vi "诊断标定3 - 副本.vi"(8 "CAN端口":u16(ring), 9 "设备索引号":u16(ring), 10 "CAN卡类型":u32(ring)=21) -> ()   [LabVIEW 2013] (continued)
            tunnel: w99 -> [_ w107]
            frame #0 {
              n49 = case shown="假" w102 {
                tunnel: w101 -> [w104 _]
                frame False {
                  n50 = Build Array("文件格式错误") -> (w105:string[])
                  n51 = call "表格编辑.vi"("新元素/子数组"=w105, "活动单元格:单元格背景色"=u32 16711680, "MCListbox引用句柄"=w104) -> ()  [unwired: 9 out]
                }
                frame True {
                }
              }
            }
            frame #1 {
              n52 = case shown="假" w107 {
                tunnel: w108 -> [w110 _]
                frame False {
                  n53 = Build Array("文件MD5码验证错误") -> (w111:string[])
                  n54 = call "表格编辑.vi"("新元素/子数组"=w111, "活动单元格:单元格背景色"=u32 16711680, "MCListbox引用句柄"=w110) -> ()  [unwired: 9 out]
                }
                frame True {
                }
              }
            }
          }
          n55 = call <vilib>:"Unset Busy.vi"() -> ()  [unwired: 11 in, 1 out]
        }
        frame True {
          n56 = stacked-sequence {
            seq-local: [w119 _ _ _] -> [_ w347 w441 _]
            seq-local: [w117 _ _ _] -> [_ w325 _ _]
            tunnel: w114 -> [w115 _ _ _]
            tunnel: w113 -> [w132 _ _ w468]
            frame #0 {
              w116 = string[][] []
              w129 = "总信息" ("section")
              n57 = local write "路径"(w115) -> ()
              n58 = call <vilib>:"Open Config Data.vi"("create file if necessary (T)"=FALSE, "configuration file path"=w115) -> ("error out"=w120:errorcluster, "refnum"=w119:T19)  [unwired: 7 in, 1 out]
              n59 = call <vilib>:"Get Key Names.vi"("section"=w129, "error in (no error)"=w120, "refnum"=w119) -> ("key names"=w128:string[], "refnum out"=w130:T19)  [unwired: 5 in, 2 out]
              n60 = for {
                tunnel: w130 -> [w136]
                tunnel: w129 -> [w135]
                tunnel: w128 -> [w134] mode=indexing
                tunnel: [w133] -> w125 mode=indexing
                n61 = call-poly <vilib>:"Read Key.vi"("section"=w135, "key"=w134, "refnum"=w136) -> ("value"=w133:string)  [unwired: 5 in, 3 out]
              }
              n62 = Index Array(array=w125) -> (element #1=w118:string, element #2=w123:string)  [unwired: 2 in]
              n63 = Decimal String To Number(string=w118) -> (number=w117:i32)  [unwired: 2 in, 1 out]
              n64 = Concatenate Strings("正在读取" ("字符串"), w123, "的配置文件" ("字符串")) -> (w121:string)
              n65 = Build Array(w121) -> (w126:string[])
              n66 = call "表格编辑.vi"("新元素/子数组"=w126, "活动单元格:单元格背景色"=u32 6618880, "MCListbox引用句柄"=w132) -> ()  [unwired: 9 out]
              n67 = local write "项目信息"(w116) -> ()
              n68 = local write "项目信息 2"(w116) -> ()
            }
            frame #1 {
              w307 = 20 ("长度")
              w348 = "主板" ("section")
              n69 = call <vilib>:"Get Key Names.vi"("section"=w348, "refnum"=w347) -> ("key names"=w149:string[], "refnum out"=w349:T19)  [unwired: 6 in, 2 out]
              n70 = for {
                tunnel: w349 -> [w361]
                tunnel: w348 -> [w360]
                tunnel: w149 -> [w359] mode=indexing
                tunnel: [w358] -> w148 mode=indexing
                n71 = call-poly <vilib>:"Read Key.vi"("section"=w360, "key"=w359, "refnum"=w361) -> ("value"=w358:string)  [unwired: 5 in, 3 out]
              }
              n72 = Search 1D Array(1D array=w149, element="总电压过高一级" ("元素"), start index (0)=0 ("开始索引(0)")) -> (index of element=w229:i32)
              n73 = Search 1D Array(1D array=w149, element="风机开启温度" ("元素"), start index (0)=w229) -> (index of element=w220:i32)
              n74 = Search 1D Array(1D array=w149, element="电池串联" ("元素"), start index (0)=w220) -> (index of element=w218:i32)
              n75 = Decrement(x=w229) -> (x-1=w346:i32)
              n76 = Array Subset(array=w149, index=1 ("索引"), length=w346) -> (w194:string[])
              n77 = Array Subset(array=w148, index=1 ("索引"), length=w346) -> (w191:string[])
              n78 = Delete From Array(array=w191, length=7 ("长度"), index=0 ("索引")) -> (deleted portion=w188:string[], array with subset deleted=w138:string[])
              n79 = Delete From Array(array=w194, length=7 ("长度"), index=0 ("索引")) -> (array with subset deleted=w147:string[])  [unwired: 1 out]
              n80 = Search 1D Array(1D array=w149, element="分流器型号" ("元素")) -> (index of element=w152:i32)  [unwired: 1 in]
              n81 = Index Array(array=w148, index=0 ("索引")) -> (element=w322:string)
              n82 = Decimal String To Number(string=w322) -> (number=w139:i32)  [unwired: 2 in, 1 out]
              n83 = Search 1D Array(1D array=w147, element="主板电池节数" ("元素")) -> (index of element=w313:i32)  [unwired: 1 in]
              n84 = Search 1D Array(1D array=w147, element="主板温度起始值" ("元素")) -> (index of element=w310:i32)  [unwired: 1 in]
              n85 = Search 1D Array(1D array=w147, element="第一个保险通道" ("元素")) -> (index of element=w309:i32)  [unwired: 1 in]
              n86 = Search 1D Array(1D array=w147, element="主板温度个数" ("元素")) -> (index of element=w311:i32)  [unwired: 1 in]
              n87 = Search 1D Array(1D array=w147, element="主板电压起始值" ("元素")) -> (index of element=w312:i32)  [unwired: 1 in]
              n88 = Search 1D Array(1D array=w147, element="第1通道电压个数" ("元素")) -> (index of element=w308:i32)  [unwired: 1 in]
              n89 = Index Array(array=w148, index=w152) -> (element=w151:string)
              n90 = for {
                N: 4 -> [_]
                tunnel: w188 -> [w357] mode=indexing
                tunnel: [w356] -> w337 mode=indexing
                n91 = Fract/Exp String To Number(string=w357) -> (number=w356:dbl)  [unwired: 3 in, 1 out]
              }
              n92 = Increment(x=w139) -> (x+1=w321:i32)
              n93 = Increment(x=w139) -> (x+1=w306:i32)
              n94 = Increment(x=w139) -> (x+1=w319:i32)
              n95 = Increment(x=w139) -> (x+1=w320:i32)
              n96 = global write "读配置文件全局.vi" "从板个数"(w139) -> ()
              n97 = local write "从板个数"(w139) -> ()
              n98 = Decimal String To Number(string=w151) -> (number=w150:i32)  [unwired: 2 in, 1 out]
              n99 = Index Array(array=w188, index #1=4 ("索引"), index #2=5 ("索引"), index #3=6 ("索引")) -> (element #1=w328:string, element #2=w327:string, element #3=w326:string)
              n100 = Index Array(array=w337) -> (element #1=w335:dbl, element #2=w334:dbl, element #3=w333:dbl, element #4=w332:dbl)  [unwired: 4 in]
              n101 = global write "EV05全局变量1.vi" "分流器型号"(w150) -> ()
              n102 = Array Subset(array=w138, index=w313, length=w321) -> (w305:string[])
              n103 = Array Subset(array=w138, index=w312, length=w320) -> (w303:string[])
              n104 = Array Subset(array=w138, index=w311, length=w319) -> (w302:string[])
              n105 = Array Subset(array=w138, index=w310, length=w306) -> (w301:string[])
              n106 = Array Subset(array=w138, index=w309, length=20 ("长度")) -> (w300:string[])
              n107 = Array Subset(array=w138, index=w308, length=w307) -> (w304:string[])
              n108 = Multiply(x=w139, y=2) -> (x*y=w140:i32)
              n109 = control-ref of="项目信息2"() -> (w340:refnum<vi>)
              n110 = Array Subset(array=w138, index=0 ("索引"), length=w140) -> (w137:string[])
              n111 = Insert Into Array(array=w305, new element #1=w304, new element #2=w303, new element #3=w302, new element #4=w301, new element #5=w300) -> ()  [unwired: 1 in, 1 out]
              n112 = property class="Clust (严格)"(reference=w340) -> (reference out=w338:refnum<vi>, "Value"=w339:T9)  [unwired: 1 in, 1 out]
              n113 = Multiply(x=w139, y=2) -> (x*y=w144:i32)
              n114 = Array Subset(array=w147, index=w313, length=w306) -> (w178:string[])
              n115 = Array Subset(array=w147, index=w312, length=w306) -> (w176:string[])
              n116 = Array Subset(array=w147, index=w311, length=w306) -> (w175:string[])
              n117 = Array Subset(array=w147, index=w310) -> (w174:string[])  [unwired: 1 in]
              n118 = Array Subset(array=w147, index=w309, length=w307) -> (w173:string[])
              n119 = Array Subset(array=w147, index=w308, length=w307) -> (w177:string[])
              n120 = Array Subset(array=w147, index=0 ("索引"), length=w144) -> (w143:string[])
              n121 = global write "读配置文件全局.vi" "表格输入"(w137) -> ()
              n122 = Build Array(w143, w137) -> (w299:string[][])
              n123 = Bundle(cluster=w339, "电池额定容量(A)"=w335, "使用者"=w325, "电池实际容量(A)"=w334, "车架(牌)号"=w327, "配置文件版本"=w326, "SOH(%)"=w332, "SOC(%)"=w333, "产品编号"=w328) -> (w165:T9)  [unwired: 1 in]
              n124 = Transpose 2D Array(2D array=w299) -> (transposed array=w166:string[][])
              n125 = Multiply(x=w139, y=4) -> (x*y=w170:i32)
              n126 = Insert Into Array(array=w178, new element #1=w177, new element #2=w176, new element #3=w175, new element #4=w174, new element #5=w173) -> (w172:string[])  [unwired: 1 in]
              n127 = Add(x=w170, y=44) -> (x+y=w168:i32)
              n128 = local write "项目信息"(w166) -> ()
              n129 = property class="Clust (严格)"(reference=w338, "Value"=w165) -> ()  [unwired: 1 in, 2 out]
              n130 = global write "读配置文件全局.vi" "项目信息"(w165) -> ()
              n131 = Array Subset(array=w148, index=w218, length=15 ("长度")) -> (w156:string[])
              n132 = Array Subset(array=w172, index=0 ("索引"), length=w168) -> ()  [unwired: 1 out]
              n133 = Array Subset(array=w148, index=w220, length=15 ("长度")) -> (w225:string[])
              n134 = Delete From Array(array=w156, length=4 ("长度"), index=6 ("索引")) -> (deleted portion=w212:string[], array with subset deleted=w211:string[])
              n135 = for {
                tunnel: w225 -> [w353] mode=indexing
                tunnel: [w352] -> w224 mode=indexing
                n136 = Fract/Exp String To Number(string=w353) -> (number=w352:dbl)  [unwired: 3 in, 1 out]
              }
              n137 = for {
                tunnel: w211 -> [w351] mode=indexing
                tunnel: [w350] -> w210 mode=indexing
                n138 = Fract/Exp String To Number(string=w351) -> (number=w350:dbl)  [unwired: 3 in, 1 out]
              }
              n139 = Array Subset(array=w148, index=w229, length=51 ("长度")) -> (w298:string[])
              n140 = for {
                tunnel: w298 -> [w355] mode=indexing
                tunnel: [w354] -> w297 mode=indexing
                n141 = Fract/Exp String To Number(string=w355) -> (number=w354:dbl)  [unwired: 3 in, 1 out]
              }
              n142 = Index Array(array=w210) -> (element #1=w205:dbl, element #2=w204:dbl, element #3=w203:dbl, element #4=w202:dbl, element #5=w201:dbl, element #6=w200:dbl, element #7=w199:dbl, element #8=w198:dbl, element #9=w197:dbl, element #10=w196:dbl, element #11=w195:dbl)  [unwired: 11 in]
              n143 = Delete From Array(array=w224, length=7 ("长度"), index=0 ("索引")) -> (deleted portion=w161:dbl[], array with subset deleted=w222:dbl[])
              n144 = Delete From Array(array=w297, length=17 ("长度"), index=0 ("索引")) -> (deleted portion=w158:dbl[], array with subset deleted=w294:dbl[])
              n145 = Array To Cluster(array=w161) -> (cluster=w223:T20)
              n146 = global write "读配置文件全局.vi" "加热控制参数"(w161) -> ()
              n147 = Index Array(array=w222) -> (element #1=w186:dbl, element #2=w185:dbl, element #3=w184:dbl, element #4=w183:dbl, element #5=w182:dbl, element #6=w181:dbl, element #7=w180:dbl, element #8=w179:dbl)  [unwired: 8 in]
              n148 = Delete From Array(array=w294, length=17 ("长度"), index=0 ("索引")) -> (deleted portion=w157:dbl[], array with subset deleted=w154:dbl[])
              n149 = Index Array(array=w212) -> (element #1=w209:string, element #2=w208:string, element #3=w206:string, element #4=w207:string)  [unwired: 4 in]
              n150 = local write "加热控制参数"(w223) -> ()
              n151 = global write "读配置文件全局.vi" "一级故障"(w158) -> ()
              n152 = local read "一级故障 5"() -> (w187:T12)
              n153 = control-ref of="电池信息"() -> (w216:refnum<vi>)
              n154 = global write "读配置文件全局.vi" "二级故障"(w157) -> ()
              n155 = global write "读配置文件全局.vi" "三级故障"(w154) -> ()
              n156 = Bundle(cluster=w187, "最大允许单体电压"=w186, "最大允许总电压"=w182, "最小允许单体电压"=w185, "最大允许充电电流"=w184, "最小允许充电电流"=w183, "最大允许充电温度"=w181, "最小允许充电温度"=w180, "电流步长"=w179) -> (w160:T12)
              n157 = property class="Clust (严格)"(reference=w216) -> (reference out=w217:refnum<vi>, "Value"=w215:T13)  [unwired: 1 in, 1 out]
              n158 = Bundle(cluster=w215, "电池串联"=w205, "电池并联"=w204, "累计放电总安时"=w198, "电池包额定容量"=w203, "电池包额定能量(kWh)"=w202, "电池包额定总电压"=w201, "累计充电总安时"=w199, "电池充满次数"=w196, "电池放空次数"=w197, "电池充电次数"=w195, "电池生产日期"=w206, "电池厂家"=w209, "电池类型"=w208, "电池包组号"=w207, "实际容量"=w200) -> (w155:T13)  [unwired: 2 in]
              n159 = Cluster To Array(cluster=w160) -> (array=w159:dbl[])
              n160 = local write "一级故障 5"(w160) -> ()
              n161 = global write "读配置文件全局.vi" "充电控制参数"(w159) -> ()
              n162 = Index Array(array=w158) -> (element #1=w287:dbl, element #2=w286:dbl, element #3=w285:dbl, element #4=w284:dbl, element #5=w283:dbl, element #6=w282:dbl, element #7=w281:dbl, element #8=w280:dbl, element #9=w279:dbl, element #10=w278:dbl, element #11=w277:dbl, element #12=w276:dbl, element #13=w275:dbl, element #14=w274:dbl, element #15=w273:dbl, element #16=w272:dbl, element #17=w271:dbl)  [unwired: 17 in]
              n163 = global write "读配置文件全局.vi" "电池信息"(w155) -> ()
              n164 = Index Array(array=w157) -> (element #1=w254:dbl, element #2=w255:dbl, element #3=w256:dbl, element #4=w257:dbl, element #5=w258:dbl, element #6=w259:dbl, element #7=w260:dbl, element #8=w261:dbl, element #9=w262:dbl, element #10=w263:dbl, element #11=w264:dbl, element #12=w265:dbl, element #13=w266:dbl, element #14=w267:dbl, element #15=w268:dbl, element #16=w269:dbl, element #17=w270:dbl)  [unwired: 17 in]
              n165 = Index Array(array=w154) -> (element #1=w249:dbl, element #2=w248:dbl, element #3=w247:dbl, element #4=w246:dbl, element #5=w245:dbl, element #6=w244:dbl, element #7=w243:dbl, element #8=w242:dbl, element #9=w241:dbl, element #10=w240:dbl, element #11=w239:dbl, element #12=w238:dbl, element #13=w237:dbl, element #14=w236:dbl, element #15=w235:dbl, element #16=w234:dbl, element #17=w233:dbl)  [unwired: 17 in]
              n166 = control-ref of="一级故障 3"() -> (w232:refnum<vi>)
              n167 = control-ref of="一级故障 2"() -> (w251:refnum<vi>)
              n168 = property class="Clust (严格)"(reference=w251) -> (reference out=w253:refnum<vi>, "Value"=w252:T10)  [unwired: 1 in, 1 out]
              n169 = property class="Clust (严格)"(reference=w232) -> (reference out=w231:refnum<vi>, "Value"=w250:T10)  [unwired: 1 in, 1 out]
              n170 = property class="Clust (严格)"(reference=w217, "Value"=w155) -> ()  [unwired: 1 in, 2 out]
              n171 = Bundle(cluster=w252, "总电压过高"=w254, "整组电压不均衡"=w258, "SOC过高"=w266, "单体电压过高"=w262, "总电压过低"=w255, "温度过高"=w256, "温度过低"=w257, "单组电压不均衡"=w259, "整组温度不均衡"=w260, "单组温度不均衡"=w261, "单体电压过低"=w263, "充电电流过高"=w264, "放电电流过高"=w265, "SOC过低"=w267, "内阻过大"=w268, "极柱温度过高"=w269, "SOH过低"=w270) -> (w163:T10)
              n172 = Bundle(cluster=w250, "总电压过高"=w249, "整组电压不均衡"=w245, "SOC过高"=w237, "单体电压过高"=w241, "总电压过低"=w248, "温度过高"=w247, "温度过低"=w246, "单组电压不均衡"=w244, "整组温度不均衡"=w243, "单组温度不均衡"=w242, "单体电压过低"=w240, "充电电流过高"=w239, "放电电流过高"=w238, "SOC过低"=w236, "内阻过大"=w235, "极柱温度过高"=w234, "SOH过低"=w233) -> (w162:T10)
              n173 = control-ref of="一级故障"() -> (w290:refnum<vi>)
              n174 = property class="Clust (严格)"(reference=w290) -> (reference out=w288:refnum<vi>, "Value"=w289:T10)  [unwired: 1 in, 1 out]
              n175 = Bundle(cluster=w289, "总电压过高"=w287, "整组电压不均衡"=w283, "SOC过高"=w275, "单体电压过高"=w279, "总电压过低"=w286, "温度过高"=w285, "温度过低"=w284, "单组电压不均衡"=w282, "整组温度不均衡"=w281, "单组温度不均衡"=w280, "单体电压过低"=w278, "充电电流过高"=w277, "放电电流过高"=w276, "SOC过低"=w274, "内阻过大"=w273, "极柱温度过高"=w272, "SOH过低"=w271) -> (w164:T10)
              n176 = property class="Clust (严格)"(reference=w288, "Value"=w164) -> ()  [unwired: 1 in, 2 out]
              n177 = property class="Clust (严格)"(reference=w253, "Value"=w163) -> ()  [unwired: 1 in, 2 out]
              n178 = property class="Clust (严格)"(reference=w231, "Value"=w162) -> ()  [unwired: 1 in, 2 out]
            }
            frame #2 {
              w426 = 1 ("索引")
              # "均衡计算-电压高阀值1级"
              n179 = call <vilib>:"Get Section Names.vi"("refnum"=w441) -> ("section names"=w442:string[], "refnum out"=w446:T19)  [unwired: 8 in, 1 out]
              n180 = local read "从板号"() -> (w424:u8)
              n181 = Delete From Array(array=w442, length=2 ("长度"), index=0 ("索引")) -> (array with subset deleted=w445:string[])  [unwired: 1 out]
              n182 = for {
                tunnel: w445 -> [w462] mode=indexing
                tunnel: w446 -> [w463]
                tunnel: [w455] -> w423 mode=indexing
                tunnel: [w454] -> w367
                n183 = call <vilib>:"Get Key Names.vi"("section"=w462, "refnum"=w463) -> ("key names"=w454:string[], "refnum out"=w461:T19)  [unwired: 6 in, 2 out]
                n184 = for {
                  tunnel: w454 -> [w467] mode=indexing
                  tunnel: w462 -> [w466]
                  tunnel: w461 -> [w465]
                  tunnel: [w464] -> w455 mode=indexing
                  n185 = call-poly <vilib>:"Read Key.vi"("section"=w466, "key"=w467, "refnum"=w465) -> ("value"=w464:string)  [unwired: 5 in, 3 out]
                }
                n186 = Index Array(array=w455, index=0 ("索引")) -> (element=w458:string)
                n187 = local read "输出数组"() -> (w459:string[][])
                n188 = Decimal String To Number(string=w458) -> (number=w457:i32)  [unwired: 2 in, 1 out]
                n189 = Decrement(x=w457) -> (x-1=w453:i32)
                n190 = Replace Array Subset(array=w459, new element=w455, index (col)=w453) -> (w456:string[][])  [unwired: 1 in]
                n191 = local write "输出数组"(w456) -> ()
              }
              "key names" <- w367
              n192 = Decrement(x=w424) -> (x-1=w440:u8)
              n193 = Index Array(array=w423, index (row)=w440) -> (element=w366:string[])  [unwired: 1 in]
              n194 = Search 1D Array(1D array=w367, element="风机开启温度" ("元素")) -> (index of element=w429:i32)  [unwired: 1 in]
              n195 = Search 1D Array(1D array=w367, element="电压过高一级" ("元素"), start index (0)=w429) -> (index of element=w392:i32)
              n196 = Search 1D Array(1D array=w367, element="均衡计算-电压高阀值1级" ("元素"), start index (0)=w392) -> (index of element=w390:i32)
              n197 = Array Subset(array=w366, index=w390, length=17 ("长度")) -> (w389:string[])
              n198 = Decrement(x=w429) -> (x-1=w427:i32)
              n199 = Array Subset(array=w366, index=w426, length=w427) -> (w364:string[])
              n200 = Array Subset(array=w366, index=w392, length=21 ("长度")) -> (w438:string[])
              n201 = Array Subset(array=w367, index=w426, length=w427) -> (w403:string[])
              n202 = Index Array(array=w366, index=0 ("索引")) -> (element=w398:string)
              n203 = Array Subset(array=w366, index=w429, length=7 ("长度")) -> (w432:string[])
              n204 = for {
                tunnel: w389 -> [w448] mode=indexing
                tunnel: [w447] -> w388 mode=indexing
                n205 = Fract/Exp String To Number(string=w448) -> (number=w447:dbl)  [unwired: 3 in, 1 out]
              }
              n206 = for {
                tunnel: w438 -> [w450] mode=indexing
                tunnel: [w449] -> w439 mode=indexing
                n207 = Fract/Exp String To Number(string=w450) -> (number=w449:dbl)  [unwired: 3 in, 1 out]
              }
              n208 = Decimal String To Number(string=w398) -> (number=w397:i32)  [unwired: 2 in, 1 out]
              n209 = for {
                tunnel: w432 -> [w452] mode=indexing
                tunnel: [w451] -> w400 mode=indexing
                n210 = Fract/Exp String To Number(string=w452) -> (number=w451:dbl)  [unwired: 3 in, 1 out]
              }
              n211 = global write "读配置文件全局2.vi" "从板板号"(w397) -> ()
              n212 = Delete From Array(array=w439, length=7 ("长度"), index=0 ("索引")) -> (deleted portion=w402:dbl[], array with subset deleted=w435:dbl[])
              n213 = Array To Cluster(array=w400) -> (cluster=w422:T20)
              n214 = global write "读配置文件全局2.vi" "加热控制参数"(w400) -> ()
              n215 = Delete From Array(array=w435, length=7 ("长度"), index=0 ("索引")) -> (deleted portion=w395:dbl[], array with subset deleted=w396:dbl[])
              n216 = local write "加热控制参数"(w422) -> ()
              n217 = Array To Cluster(array=w402) -> (cluster=w406:T20)
              n218 = Array To Cluster(array=w396) -> (cluster=w404:T20)
              n219 = Array To Cluster(array=w395) -> (cluster=w405:T20)
              n220 = global write "读配置文件全局2.vi" "三级故障阀值"(w396) -> ()
              n221 = global write "读配置文件全局2.vi" "一级故障阀值"(w402) -> ()
              n222 = global write "读配置文件全局2.vi" "二级故障阀值"(w395) -> ()
              n223 = local write "一级故障 6"(w406) -> ()
              n224 = local write "一级故障 8"(w404) -> ()
              n225 = local write "一级故障 7"(w405) -> ()
              n226 = Search 1D Array(1D array=w403, element="第1通道电压个数" ("元素")) -> (index of element=w414:i32)  [unwired: 1 in]
              n227 = Search 1D Array(1D array=w403, element="电压个数" ("元素")) -> ()  [unwired: 1 in, 1 out]
              n228 = Search 1D Array(1D array=w403, element="温度个数" ("元素")) -> (index of element=w416:i32)  [unwired: 1 in]
              n229 = Search 1D Array(1D array=w403, element="第一个保险通道" ("元素")) -> (index of element=w415:i32)  [unwired: 1 in]
              n230 = Array Subset(array=w364, length=2 ("长度")) -> (w411:string[])  [unwired: 1 in]
              n231 = Array Subset(array=w364, index=w416, length=2 ("长度")) -> (w409:string[])
              n232 = Array Subset(array=w364, index=w415, length=20 ("长度")) -> (w408:string[])
              n233 = Array Subset(array=w364, index=w414, length=20 ("长度")) -> (w410:string[])
              n234 = Array Subset(array=w364, length=27 ("长度")) -> (w363:string[])  [unwired: 1 in]
              n235 = Insert Into Array(array=w411, new element #1=w410, new element #2=w409, new element #3=w408) -> ()  [unwired: 1 in, 1 out]
              n236 = Build Array(string[] ["电压个数", "温度个数", "第一个保险通道", "第一个保险位置", "第二个保险通道", "第二个保险位置", "第三个保险通道", "第三个保险位置", "第四个保险通道", "第四个保险位置", "第五个保险通道", "第五个保险位置", "第六个保险通道", "第六个保险位置", "第七个保险通道", "第七个保险位置", "第八个保险通道", "第八个保险位置", "第九个保险通道", "第九个保险位置", "第十个保险通道", "第十个保险位置", "第1通道电压个数", "第2通道电压个数", "第3通道电压个数", "第4通道电压个数", "第5通道电压个数"], w363) -> (w407:string[][])
              n237 = global write "读配置文件全局2.vi" "表格"(w363) -> ()
              n238 = Index Array(array=w388) -> (element #1=w385:dbl, element #2=w384:dbl, element #3=w383:dbl, element #4=w382:dbl, element #5=w381:dbl, element #6=w380:dbl, element #7=w379:dbl, element #8=w378:dbl, element #9=w377:dbl, element #10=w376:dbl, element #11=w375:dbl, element #12=w374:dbl, element #13=w373:dbl, element #14=w372:dbl, element #15=w371:dbl, element #16=w370:dbl, element #17=w369:dbl, element #18=w368:dbl)  [unwired: 18 in]
              n239 = Transpose 2D Array(2D array=w407) -> (transposed array=w401:string[][])
              n240 = local write "项目信息 2"(w401) -> ()
              n241 = local read "均衡参数"() -> (w387:T17)
              n242 = Bundle(cluster=w387, "充电结束电压(90%)"=w378, "充电结束电压(91%)"=w377, "充电结束电压(92%)"=w376, "充电结束电压(93%)"=w375, "充电结束电压(94%)"=w374, "均衡计算-电压高阀值1级"=w385, "均衡计算-电压高阀值2级"=w384, "均衡计算-电压低阀值1级"=w383, "均衡计算-电压低阀值2级"=w382, "均衡计算-最低电压阀值"=w381, "均衡停止-最低电压阀值"=w380, "均衡计算-电压极差阀值"=w379, "充电结束电压(95%)"=w373, "充电结束电压(96%)"=w372, "充电结束电压(97%)"=w371, "充电结束电压(98%)"=w370, "充电结束电压(99%)"=w369, "充电结束电压(100%)"=w368) -> (w386:T17)
              n243 = local write "均衡参数"(w386) -> ()
            }
            frame #3 {
              n244 = call <vilib>:"Unset Busy.vi"() -> ()  [unwired: 11 in, 1 out]
              n245 = Build Array("读取完成") -> (w471:string[])
              n246 = property on="全部写入" class="Bool (严格)"("DisabledEnum"=0) -> ()  [unwired: 2 in, 2 out]
              n247 = call "表格编辑.vi"("新元素/子数组"=w471, "活动单元格:单元格背景色"=u32 6618880, "MCListbox引用句柄"=w468) -> ()  [unwired: 9 out]
            }
          }
        }
      }
    }
  }
  n248 = stacked-sequence {
    frame #0 {
    }
  }
  n249 = stacked-sequence {
    tunnel: [w485] -> w31
    frame #0 {
      w478 = 1
      w479 = string[][] []
      w498 = string[] ["", "", "", "", "", "", "", "", "", "", "", "", "", "", "", "", "", "", "", "", "", "", "", "", "", "", "", "", "", "", "", ""]
      w497 = string[][] [["", "", "", "", "", "", "", "", "", "", "", "", "", "", "", "", "", "", "", "", "", "", "", "", "", "", "", "", "", "", "", "", "", "", "", "", "", "", "", "", ""], ["", "", "", "", "", "", "", "", "", "", "", "", "", "", "", "", "", "", "", "", "", "", "", "", "", "", "", "", "", "", "", "", "", "", "", "", "", "", "", "", ""], ["", "", "", "", "", "", "", "", "", "", "", "", "", "", "", "", "", "", "", "", "", "", "", "", "", "", "", "", "", "", "", "", "", "", "", "", "", "", "", "", ""], ["", "", "", "", "", "", "", "", "", "", "", "", "", "", "", "", "", "", "", "", "", "", "", "", "", "", "", "", "", "", "", "", "", "", "", "", "", "", "", "", ""], ["", "", "", "", "", "", "", "", "", "", "", "", "", "", "", "", "", "", "", "", "", "", "", "", "", "", "", "", "", "", "", "", "", "", "", "", "", "", "", "", ""], ["", "", "", "", "", "", "", "", "", "", "", "", "", "", "", "", "", "", "", "", "", "", "", "", "", "", "", "", "", "", "", "", "", "", "", "", "", "", "", "", ""], ["", "", "", "", "", "", "", "", "", "", "", "", "", "", "", "", "", "", "", "", "", "", "", "", "", "", "", "", "", "", "", "", "", "", "", "", "", "", "", "", ""], ["", "", "", "", "", "", "", "", "", "", "", "", "", "", "", "", "", "", "", "", "", "", "", "", "", "", "", "", "", "", "", "", "", "", "", "", "", "", "", "", ""], ["", "", "", "", "", "", "", "", "", "", "", "", "", "", "", "", "", "", "", "", "", "", "", "", "", "", "", "", "", "", "", "", "", "", "", "", "", "", "", "", ""], ["", "", "", "", "", "", "", "", "", "", "", "", "", "", "", "", "", "", "", "", "", "", "", "", "", "", "", "", "", "", "", "", "", "", "", "", "", "", "", "", ""], ["", "", "", "", "", "", "", "", "", "", "", "", "", "", "", "", "", "", "", "", "", "", "", "", "", "", "", "", "", "", "", "", "", "", "", "", "", "", "", "", ""], ["", "", "", "", "", "", "", "", "", "", "", "", "", "", "", "", "", "", "", "", "", "", "", "", "", "", "", "", "", "", "", "", "", "", "", "", "", "", "", "", ""], ["", "", "", "", "", "", "", "", "", "", "", "", "", "", "", "", "", "", "", "", "", "", "", "", "", "", "", "", "", "", "", "", "", "", "", "", "", "", "", "", ""], ["", "", "", "", "", "", "", "", "", "", "", "", "", "", "", "", "", "", "", "", "", "", "", "", "", "", "", "", "", "", "", "", "", "", "", "", "", "", "", "", ""], ["", "", "", "", "", "", "", "", "", "", "", "", "", "", "", "", "", "", "", "", "", "", "", "", "", "", "", "", "", "", "", "", "", "", "", "", "", "", "", "", ""], ["", "", "", "", "", "", "", "", "", "", "", "", "", "", "", "", "", "", "", "", "", "", "", "", "", "", "", "", "", "", "", "", "", "", "", "", "", "", "", "", ""], ["", "", "", "", "", "", "", "", "", "", "", "", "", "", "", "", "", "", "", "", "", "", "", "", "", "", "", "", "", "", "", "", "", "", "", "", "", "", "", "", ""], ["", "", "", "", "", "", "", "", "", "", "", "", "", "", "", "", "", "", "", "", "", "", "", "", "", "", "", "", "", "", "", "", "", "", "", "", "", "", "", "", ""], ["", "", "", "", "", "", "", "", "", "", "", "", "", "", "", "", "", "", "", "", "", "", "", "", "", "", "", "", "", "", "", "", "", "", "", "", "", "", "", "", ""], ["", "", "", "", "", "", "", "", "", "", "", "", "", "", "", "", "", "", "", "", "", "", "", "", "", "", "", "", "", "", "", "", "", "", "", "", "", "", "", "", ""], ["", "", "", "", "", "", "", "", "", "", "", "", "", "", "", "", "", "", "", "", "", "", "", "", "", "", "", "", "", "", "", "", "", "", "", "", "", "", "", "", ""], ["", "", "", "", "", "", "", "", "", "", "", "", "", "", "", "", "", "", "", "", "", "", "", "", "", "", "", "", "", "", "", "", "", "", "", "", "", "", "", "", ""], ["", "", "", "", "", "", "", "", "", "", "", "", "", "", "", "", "", "", "", "", "", "", "", "", "", "", "", "", "", "", "", "", "", "", "", "", "", "", "", "", ""], ["", "", "", "", "", "", "", "", "", "", "", "", "", "", "", "", "", "", "", "", "", "", "", "", "", "", "", "", "", "", "", "", "", "", "", "", "", "", "", "", ""], ["", "", "", "", "", "", "", "", "", "", "", "", "", "", "", "", "", "", "", "", "", "", "", "", "", "", "", "", "", "", "", "", "", "", "", "", "", "", "", "", ""], ["", "", "", "", "", "", "", "", "", "", "", "", "", "", "", "", "", "", "", "", "", "", "", "", "", "", "", "", "", "", "", "", "", "", "", "", "", "", "", "", ""], ["", "", "", "", "", "", "", "", "", "", "", "", "", "", "", "", "", "", "", "", "", "", "", "", "", "", "", "", "", "", "", "", "", "", "", "", "", "", "", "", ""], ["", "", "", "", "", "", "", "", "", "", "", "", "", "", "", "", "", "", "", "", "", "", "", "", "", "", "", "", "", "", "", "", "", "", "", "", "", "", "", "", ""], ["", "", "", "", "", "", "", "", "", "", "", "", "", "", "", "", "", "", "", "", "", "", "", "", "", "", "", "", "", "", "", "", "", "", "", "", "", "", "", "", ""], ["", "", "", "", "", "", "", "", "", "", "", "", "", "", "", "", "", "", "", "", "", "", "", "", "", "", "", "", "", "", "", "", "", "", "", "", "", "", "", "", ""], ["", "", "", "", "", "", "", "", "", "", "", "", "", "", "", "", "", "", "", "", "", "", "", "", "", "", "", "", "", "", "", "", "", "", "", "", "", "", "", "", ""], ["", "", "", "", "", "", "", "", "", "", "", "", "", "", "", "", "", "", "", "", "", "", "", "", "", "", "", "", "", "", "", "", "", "", "", "", "", "", "", "", ""], ["", "", "", "", "", "", "", "", "", "", "", "", "", "", "", "", "", "", "", "", "", "", "", "", "", "", "", "", "", "", "", "", "", "", "", "", "", "", "", "", ""], ["", "", "", "", "", "", "", "", "", "", "", "", "", "", "", "", "", "", "", "", "", "", "", "", "", "", "", "", "", "", "", "", "", "", "", "", "", "", "", "", ""], ["", "", "", "", "", "", "", "", "", "", "", "", "", "", "", "", "", "", "", "", "", "", "", "", "", "", "", "", "", "", "", "", "", "", "", "", "", "", "", "", ""], ["", "", "", "", "", "", "", "", "", "", "", "", "", "", "", "", "", "", "", "", "", "", "", "", "", "", "", "", "", "", "", "", "", "", "", "", "", "", "", "", ""], ["", "", "", "", "", "", "", "", "", "", "", "", "", "", "", "", "", "", "", "", "", "", "", "", "", "", "", "", "", "", "", "", "", "", "", "", "", "", "", "", ""], ["", "", "", "", "", "", "", "", "", "", "", "", "", "", "", "", "", "", "", "", "", "", "", "", "", "", "", "", "", "", "", "", "", "", "", "", "", "", "", "", ""], ["", "", "", "", "", "", "", "", "", "", "", "", "", "", "", "", "", "", "", "", "", "", "", "", "", "", "", "", "", "", "", "", "", "", "", "", "", "", "", "", ""], ["", "", "", "", "", "", "", "", "", "", "", "", "", "", "", "", "", "", "", "", "", "", "", "", "", "", "", "", "", "", "", "", "", "", "", "", "", "", "", "", ""], ["", "", "", "", "", "", "", "", "", "", "", "", "", "", "", "", "", "", "", "", "", "", "", "", "", "", "", "", "", "", "", "", "", "", "", "", "", "", "", "", ""]]
      w486 = TRUE
      w481 = u32 16777215
      w477 = FALSE ("判定2")
      n250 = control-ref of="结果"() -> (w482:refnum<vi>)
      n251 = control-ref of="模块软件版本 2"() -> (w483:refnum<vi>)
      n252 = control-ref of="结果"() -> (w484:refnum<vi>)
      n253 = control-ref of="单选选项2"() -> (w501:refnum<vi>)
      n254 = control-ref of="单选选项1"() -> (w502:refnum<vi>)
      n255 = local write "key names"(string[] []) -> ()
      n256 = property on="项目信息" class="Tbl (严格)"("Disabled"=w478) -> ()  [unwired: 2 in, 2 out]
      n257 = property on="电池实际容量(A)" class="DigNum (严格)"("Disabled"=w478) -> ()  [unwired: 2 in, 2 out]
      n258 = property on="使用者" class="DigNum (严格)"("Disabled"=w478) -> ()  [unwired: 2 in, 2 out]
      n259 = property on="SOH(%)" class="DigNum (严格)"("Disabled"=w478) -> ()  [unwired: 2 in, 2 out]
      n260 = property on="电池额定容量(A)" class="DigNum (严格)"("Disabled"=w478) -> ()  [unwired: 2 in, 2 out]
      n261 = local write "主从选择"(enum32{"主板", "从板"}."主板" ("主从选择")) -> ()
      n262 = property on="SOC(%)" class="DigNum (严格)"("Disabled"=w478) -> ()  [unwired: 2 in, 2 out]
      n263 = local write "等级 2"(T21."从板信息" ("等级 2")) -> ()
      n264 = local write "主板2"(T8."项目信息" ("主从板")) -> ()
      n265 = property class="MCListbox (严格)"(reference=w484, "ItemNames"=w479) -> ()  [unwired: 1 in, 2 out]
      n266 = property class="MCListbox (严格)"(reference=w483, "ItemNames"=w479) -> ()  [unwired: 1 in, 2 out]
      n267 = property class="MCListbox (严格)"(reference=w482, "ItemNames"=w479) -> ()  [unwired: 1 in, 2 out]
      n268 = property class="Bool (严格)"(reference=w501, "BoolText.TextColor"=u32 87470) -> ()  [unwired: 1 in, 2 out]
      n269 = property class="Bool (严格)"(reference=w502, "BoolText.TextColor"=w481) -> ()  [unwired: 1 in, 2 out]
      n270 = property on="从板号" class="DigNum (严格)"("NumText.BGColor"=w481) -> ()  [unwired: 2 in, 2 out]
      n271 = local write "主从板"(enum32{"单选选项2", "单选选项1"}."单选选项1" ("主从板")) -> ()
      n272 = property on="项目信息2" class="Clust (严格)"("DisabledEnum"=w478) -> ()  [unwired: 2 in, 2 out]
      n273 = property on="系统时钟" class="Str"("Disabled"=w478) -> ()  [unwired: 2 in, 2 out]
      n274 = property on="配置文件版本" class="Str"("Disabled"=w478) -> ()  [unwired: 2 in, 2 out]
      n275 = property on="车架(牌)号" class="Str"("Disabled"=w478) -> ()  [unwired: 2 in, 2 out]
      n276 = property on="产品编号" class="Str"("Disabled"=w478) -> ()  [unwired: 2 in, 2 out]
      n277 = local write "判定3"(w486) -> ()
      n278 = local write "清BUFF"(w486) -> ()
      n279 = local write "1"(w486) -> ()
      n280 = property on="从板个数" class="DigNum (严格)"("Visible"=w486) -> ()  [unwired: 2 in, 2 out]
      n281 = property on="从板个数" class="DigNum (严格)"("NumText.BGColor"=u32 16448250) -> ()  [unwired: 2 in, 2 out]
      n282 = Not(x=w486) -> (.not. x?=w505:bool)
      n283 = local write "布尔"(w486) -> ()
      n284 = property on="主板选项" class="Tree (严格)"("Visible"=w486) -> ()  [unwired: 2 in, 2 out]
      n285 = property on="全部写入" class="Bool (严格)"("DisabledEnum"=2) -> ()  [unwired: 2 in, 2 out]
      n286 = property on="从板选项" class="Tree (严格)"("Visible"=w505) -> ()  [unwired: 2 in, 2 out]
      n287 = property on="当前从板板号" class="DigNum (严格)"("Visible"=w505) -> ()  [unwired: 2 in, 2 out]
      n288 = control-ref of="结果"() -> (w492:refnum<vi>)
      n289 = control-ref of="结果"() -> (w489:refnum<vi>)
      n290 = local write "强制停止版本读取"(w477) -> ()
      n291 = local write "强制终止读写标记"(w477) -> ()
      n292 = control-ref of="项目信息"() -> (w490:refnum<vi>)
      n293 = local write "判定2"(w477) -> ()
      n294 = local write "停止"(w477) -> ()
      n295 = local write "控制1"(w477) -> ()
      n296 = local write "消除"(w477) -> ()
      n297 = global write "EV05全局变量1.vi" "授权功能"(w477) -> ()
      n298 = local write "继电器超时处理"(w477) -> ()
      n299 = local write "1 6"(w477) -> ()
      n300 = local write "1 7"(w477) -> ()
      n301 = local write "1 8"(w477) -> ()
      n302 = local write "1 9"(w477) -> ()
      n303 = local write "1 10"(w477) -> ()
      n304 = local write "1 2"(w477) -> ()
      n305 = local write "1 3"(w477) -> ()
      n306 = local write "1 4"(w477) -> ()
      n307 = local write "1 5"(w477) -> ()
      n308 = local write "1 11"(w477) -> ()
      n309 = for {
        N: 150 -> [_]
        tunnel: w492 -> [w533]
        i -> [w531]
        n310 = Bundle(w531, 0) -> (w529:cluster{i32, i32})  [unwired: 1 out]
        n311 = property class="MCListbox (严格)"(reference=w533, "ActiveCell"=w529, "CellBG"=u32 16448250) -> ()  [unwired: 1 in, 2 out]
      }
      n312 = for {
        N: 150 -> [_]
        tunnel: w490 -> [w528]
        i -> [w527]
        n313 = Bundle(w527, 0) -> (w525:cluster{i32, i32})  [unwired: 1 out]
        n314 = property class="Tbl (严格)"(reference=w528, "Active Cell"=w525, "Cell BG Color"=u32 16448250) -> ()  [unwired: 1 in, 2 out]
      }
      n315 = for {
        N: 150 -> [_]
        tunnel: w489 -> [w538]
        i -> [w536]
        n316 = Bundle(w536, 0) -> (w534:cluster{i32, i32})  [unwired: 1 out]
        n317 = property class="MCListbox (严格)"(reference=w538, "ActiveCell"=w534, "CellBG"=u32 16448250) -> ()  [unwired: 1 in, 2 out]
      }
      n318 = stacked-sequence {
        tunnel: [_ _ w512] -> w485
        frame #0 {
          w506 = u32 4 items=["PCI5121"=1, "PCI9810"=2, "USBCAN1"=3, "USBCAN2"=4, "PCI9820"=5, "PCI5110"=7, "CANLite(mini)"=8, "ISA9620"=9, "ISA5420"=10, "PC104CAN"=11, "DNP9810"=13, "PCI9840B"=14, "PC104C2"=15, "PCI9820I"=16, "pec9920"=18, "USBCAN_E_U"=20, "USBCAN_2E_U"=21] ("CAN卡类型")
          n319 = local write "CAN卡类型"(w506) -> ()
        }
        frame #1 {
          n320 = disable-structure shown="启用" {
            frame Disabled {
              n321 = local read "设备索引号"() -> (w508:u16)
              n322 = local read "CAN卡类型"() -> (w507:u32)
              n323 = local read "CAN端口"() -> (w509:u16)
              n324 = dll-call lib="PTH1mabs FBluewave New EnergySVN_WorkBMS_Monitor_Bnet01trunk参数设置data\nkerneldlls\nusbcan.dll" fn="VCI_ClearBuffer"("DeviceType"=w507, "DeviceInd"=w508, "CANInd"=w509) -> (error out=w510:errorcluster)  [unwired: 4 in, 4 out]
              n325 = call <vilib>:"Clear Errors.vi"("error in (no error)"=w510) -> ()  [unwired: 6 in, 1 out]
            }
            frame Enabled {
            }
          }
        }
        frame #2 {
          w519 = u8 0 items=["Normal", "Listen Only"] ("工作方式")
          w518 = u8 1 items=["Dual Filter", "Single Filter"] ("滤波方式")
          n326 = local read "设备索引号"() -> (w514:u16)
          n327 = local read "CAN卡类型"() -> (w513:u32)
          n328 = local read "CAN端口"() -> (w515:u16)
          n329 = call "CAN_Init-8.6.vi"("CAN卡类型"=w513, "设备索引号"=w514, "CAN端口"=w515, "操作类型"=enum16{"初始化CAN", "关闭CAN"}."初始化CAN", "滤波方式"=w518, "Accept Code"=u32 3221225472, "簇"=T23 {"打开CAN"=TRUE, "初始化CAN"=TRUE, "开始CAN"=TRUE, "重启"=FALSE, "关闭CAN"=FALSE}, "Mask Code"=u32 1073741823 ("Accept Code"), "工作方式"=w519, "是否滤波"=TRUE, "滤波选择"=T22 {"fiter_mode"=1, "fiter_endid"=402653184, "fiter_startid"=419430399}) -> ("CAN 操作结果"=→"CAN":bool, "error out"=w512:errorcluster)  [unwired: 3 in, 4 out]
        }
      }
      n330 = local write "加热继电器(从)"(w477) -> ()
      n331 = local write "风机继电器(从)"(w477) -> ()
      n332 = local write "DO1"(w477) -> ()
      n333 = local write "DO2"(w477) -> ()
      n334 = local write "DO1 2"(w477) -> ()
      n335 = local write "正级继电器"(w477) -> ()
      n336 = local write "负级继电器"(w477) -> ()
      n337 = local write "加热继电器"(w477) -> ()
      n338 = local write "充电继电器"(w477) -> ()
      n339 = local write "风机继电器"(w477) -> ()
      n340 = local write "预充电继电器"(w477) -> ()
      n341 = property on="保存版本信息" class="Bool (严格)"("Visible"=w477) -> ()  [unwired: 2 in, 2 out]
      n342 = property on="单个读取" class="Bool (严格)"("Visible"=w477) -> ()  [unwired: 2 in, 2 out]
      n343 = property on="单个写入" class="Bool (严格)"("Visible"=w477) -> ()  [unwired: 2 in, 2 out]
      n344 = local write "正级继电器 12"(w477) -> ()
      n345 = local write "正级继电器 2"(w477) -> ()
      n346 = local write "正级继电器 3"(w477) -> ()
      n347 = local write "正级继电器 4"(w477) -> ()
      n348 = local write "正级继电器 5"(w477) -> ()
      n349 = local write "正级继电器 6"(w477) -> ()
      n350 = local write "正级继电器 7"(w477) -> ()
      n351 = local write "正级继电器 8"(w477) -> ()
      n352 = local write "正级继电器 9"(w477) -> ()
      n353 = local write "正级继电器 10"(w477) -> ()
      n354 = local write "正级继电器 11"(w477) -> ()
      n355 = property on="从板号" class="DigNum (严格)"("Visible"=w477) -> ()  [unwired: 2 in, 2 out]
      "电池故障" <- w479
      "模块版本值" <- w497
      "硬件版本" <- w498
      "模块版本名称" <- w497
      "平台软件版本" <- w498
      "项目软件版本" <- w498
      "模块个数" <- u8[] [0, 0, 0, 0, 0, 0, 0, 0, 0, 0, 0, 0, 0, 0, 0, 0, 0, 0, 0, 0, 0, 0, 0, 0, 0, 0, 0, 0, 0, 0, 0, 0] ("模块个数")
    }
  }
  n356 = stacked-sequence {
    tunnel: [w539] -> w34
    frame #0 {
      n357 = call <vilib>:"Set Busy.vi"() -> ()  [unwired: 10 in, 2 out]
      n358 = disable-structure shown="禁用" {
        frame Disabled {
          n359 = control-ref of="主板选项"() -> (w658:refnum<vi>)
          n360 = stacked-sequence {
            tunnel: w658 -> [w660 w818 w856]
            frame #0 {
              # "加热和充电控制参数"
              n361 = global read "功能码全局.vi" "主板控制类信息10"() -> (w670:bool[])
              n362 = Index Array(array=w670) -> (element #5=w664:bool, element #6=w662:bool, element #7=w663:bool, element #8=w661:bool)  [unwired: 8 in, 4 out]
              n363 = Not Or(1:w663, 2:w664) -> (0:w669:bool)
              n364 = Not Or(1:w661, 2:w662) -> (0:w667:bool)
              n365 = for {
                N: 8 -> [_]
                tunnel: w660 -> [w790]
                tunnel: w669 -> [w786]
                tunnel: [w785] -> w668
                i -> [w788]
                n366 = Add(x=w788, y=69) -> (x+y=w789:i32)
                n367 = property class="Tree (严格)"(reference=w790, "Active Item Row Number"=w789, "Disabled?"=w786) -> (error out=w785:errorcluster)  [unwired: 1 in, 1 out]
              }
              n368 = for {
                N: 9 -> [_]
                tunnel: w660 -> [w784]
                tunnel: w667 -> [w780]
                tunnel: w668 -> [w779]
                tunnel: [w778] -> w659
                i -> [w782]
                n369 = Add(x=w782, y=77) -> (x+y=w783:i32)
                n370 = property class="Tree (严格)"(reference=w784, error in=w779, "Active Item Row Number"=w783, "Disabled?"=w780) -> (error out=w778:errorcluster)  [unwired: 1 out]
              }
              n371 = stacked-sequence {
                tunnel: w660 -> [w690 _ _]
                tunnel: w659 -> [w689 _ _]
                frame #0 {
                  # "电池信息"
                  n372 = global read "功能码全局.vi" "主板版本号11"() -> (w691:bool[])
                  n373 = global read "功能码全局.vi" "主板项目信息4"() -> (w673:bool[])
                  n374 = Index Array(array=w691) -> (element #1=w687:bool, element #2=w686:bool, element #3=w680:bool, element #4=w674:bool, element #6=w679:bool, element #7=w678:bool, element #8=w677:bool)  [unwired: 8 in, 1 out]
                  n375 = Index Array(array=w673, index=4 ("索引")) -> (element=w671:bool)
                  n376 = Or(x=w680, y=w674) -> (x .or. y?=w675:bool)
                  n377 = Not(x=w678) -> (.not. x?=w682:bool)
                  n378 = Not(x=w677) -> (.not. x?=w681:bool)
                  n379 = Not(x=w679) -> (.not. x?=w683:bool)
                  n380 = property on="硬件版本号" class="Str"("Visible"=w680) -> ()  [unwired: 2 in, 2 out]
                  n381 = property on="读硬件版本号" class="Bool (严格)"("Visible"=w680) -> ()  [unwired: 2 in, 2 out]
                  n382 = property on="项目软件版本号" class="Str"("Visible"=w680) -> ()  [unwired: 2 in, 2 out]
                  n383 = property on="项目软本读取" class="Bool (严格)"("Visible"=w680) -> ()  [unwired: 2 in, 2 out]
                  n384 = property on="继电器屏1 2" class="TabCtl (严格)"("Visible"=w683) -> ()  [unwired: 2 in, 2 out]
                  n385 = property on="均衡屏" class="TabCtl (严格)"("Visible"=w681) -> ()  [unwired: 2 in, 2 out]
                  n386 = property on="继电器屏1 2" class="TabCtl (严格)"("Visible"=w683) -> ()  [unwired: 2 in, 2 out]
                  n387 = property on="DO屏" class="TabCtl (严格)"("Visible"=w682) -> ()  [unwired: 2 in, 2 out]
                  n388 = Compound Arithmetic op=OR(w679, w678, w677) -> (w676:bool)
                  n389 = Not Or(1:w686, 2:w687) -> (0:w685:bool)
                  n390 = stacked-sequence {
                    tunnel: w676 -> [_ w696 _]
                    tunnel: w675 -> [_ _ w700]
                    tunnel: w671 -> [w692 _ _]
                    frame #0 {
                      n391 = case shown="真" w692 {
                        frame False {
                        }
                        frame True {
                          n392 = local write "主界面选项"(enum32{"单选选项1", "单选选项2", "单选选项2 2", "单选选项2 3"}."单选选项2 3" ("主界面选项")) -> ()
                          n393 = local write "面板选择"(T7."高压板校正" ("面板选择")) -> ()
                        }
                      }
                      n394 = control-ref of="单选选项2 3"() -> (w693:refnum<vi>)
                      n395 = property class="Bool (严格)"(reference=w693, "Visible"=w692) -> ()  [unwired: 1 in, 2 out]
                    }
                    frame #1 {
                      n396 = control-ref of="单选选项2 2"() -> (w697:refnum<vi>)
                      n397 = case shown="真" w696 {
                        frame False {
                        }
                        frame True {
                          n398 = local write "主界面选项"(enum32{"单选选项1", "单选选项2", "单选选项2 2", "单选选项2 3"}."单选选项2 2" ("主界面选项")) -> ()
                          n399 = local write "面板选择"(enum32{"读写参数", "版本读取", "其它诊断"}."其它诊断" ("选项卡控件 2")) -> ()
                        }
                      }
                      n400 = property class="Bool (严格)"(reference=w697, "Visible"=w696) -> ()  [unwired: 1 in, 2 out]
                    }
                    frame #2 {
                      n401 = control-ref of="单选选项2"() -> (w701:refnum<vi>)
                      n402 = case shown="真" w700 {
                        frame False {
                        }
                        frame True {
                          n403 = local write "主界面选项"(enum32{"单选选项1", "单选选项2", "单选选项2 2", "单选选项2 3"}."单选选项2" ("主界面选项")) -> ()
                          n404 = local write "面板选择"(enum32{"读写参数", "版本读取", "其它诊断"}."版本读取" ("选项卡控件 2")) -> ()
                        }
                      }
                      n405 = property class="Bool (严格)"(reference=w701, "Visible"=w700) -> ()  [unwired: 1 in, 2 out]
                    }
                  }
                  n406 = for {
                    N: 5 -> [_]
                    tunnel: w690 -> [w710]
                    tunnel: w685 -> [w706]
                    tunnel: w689 -> [w705]
                    tunnel: [w704] -> w688
                    i -> [w708]
                    n407 = Add(x=w708, y=86) -> (x+y=w709:i32)
                    n408 = property class="Tree (严格)"(reference=w710, error in=w705, "Active Item Row Number"=w709, "Disabled?"=w706) -> (error out=w704:errorcluster)  [unwired: 1 out]
                  }
                  n409 = property on="模块软件版本 2" class="MCListbox (严格)"("Visible"=w674) -> ()  [unwired: 2 in, 2 out]
                  n410 = property on="模块软件版本" class="Enum (严格)"("Visible"=w674) -> ()  [unwired: 2 in, 2 out]
                  n411 = property on="平台软件版本号" class="Str"("Visible"=w674) -> ()  [unwired: 2 in, 2 out]
                  n412 = property on="模块版本读取" class="Bool (严格)"("Visible"=w674) -> ()  [unwired: 2 in, 2 out]
                  n413 = property on="平台软件版本读取" class="Bool (严格)"("Visible"=w674) -> ()  [unwired: 2 in, 2 out]
                  n414 = call <vilib>:"Clear Errors.vi"("error in (no error)"=w688) -> ()  [unwired: 6 in, 1 out]
                }
                frame #1 {
                  n415 = global read "功能码全局.vi" "主板项目信息7"() -> (w750:bool[])
                  n416 = global read "功能码全局.vi" "主板控制类信息10"() -> (w746:bool[])
                  n417 = global read "功能码全局.vi" "主板故障阀值9"() -> (w749:bool[])
                  n418 = global read "功能码全局.vi" "主板项目信息4"() -> (w728:bool[])
                  n419 = global read "功能码全局.vi" "主板项目信息5"() -> (w737:bool[])
                  n420 = global read "功能码全局.vi" "主板项目信息6"() -> (w727:bool[])
                  n421 = global read "功能码全局.vi" "主板版本号11"() -> (w736:bool[])
                  n422 = Delete From Array(array=w727, length=1 ("长度"), index=0 ("索引")) -> (deleted portion=w738:bool[], array with subset deleted=w754:bool[])
                  n423 = Index Array(array=w728, index #1=5 ("索引"), index #2=6 ("索引"), index #3=7 ("索引")) -> (element #1=w739:bool, element #2=w755:bool, element #3=w711:bool)
                  n424 = Index Array(array=w736) -> (element #1=w743:bool, element #2=w759:bool)  [unwired: 2 in]
                  n425 = Array Subset(array=w749, index=2 ("索引"), length=3 ("长度")) -> (w741:bool[])
                  n426 = Delete From Array(array=w750, length=3 ("索引"), index=2 ("长度")) -> (deleted portion=w740:bool[], array with subset deleted=w756:bool[])
                  n427 = Array Subset(array=w746, index=4 ("索引"), length=2 ("长度")) -> (w742:bool[])
                  n428 = global read "功能码全局.vi" "18"() -> (w719:bool[])
                  n429 = global read "功能码全局.vi" "16"() -> (w720:bool[])
                  n430 = Insert Into Array(array=w737, new element #1=w738, new element #2=w739, new element #3=w740, new element #4=w741, new element #5=w742, new element #6=w743) -> (w760:bool[])  [unwired: 1 in]
                  n431 = Array Subset(array=w746, index=6 ("索引"), length=2 ("长度")) -> (w758:bool[])
                  n432 = Array Subset(array=w749, index=5 ("索引"), length=3 ("长度")) -> (w757:bool[])
                  n433 = And Array Elements(Boolean array=w760) -> (logical AND=w725:bool)
                  n434 = Array Subset(array=w719, index=0 ("索引"), length=8 ("长度")) -> (w717:bool[])
                  n435 = Array Subset(array=w720, index=4 ("索引"), length=4 ("长度")) -> (w716:bool[])
                  n436 = Or Array Elements(Boolean array=w760) -> (logical OR=w712:bool)
                  n437 = Insert Into Array(array=w754, new element #1=w755, new element #2=w756, new element #3=w757, new element #4=w758, new element #5=w759) -> (w761:bool[])  [unwired: 1 in]
                  n438 = property on="全部读取" class="Bool (严格)"("Visible"=w725) -> ()  [unwired: 2 in, 2 out]
                  n439 = global read "功能码全局.vi" "15"() -> (w718:bool[])
                  n440 = And Array Elements(Boolean array=w761) -> (logical AND=w726:bool)
                  n441 = property on="全部写入" class="Bool (严格)"("Visible"=w726) -> ()  [unwired: 2 in, 2 out]
                  n442 = Or Array Elements(Boolean array=w761) -> (logical OR=w762:bool)
                  n443 = Insert Into Array(array=w718, new element #1=w717, new element #2=w716) -> (w715:bool[])  [unwired: 1 in]
                  n444 = Or Array Elements(Boolean array=w715) -> (logical OR=w714:bool)
                  n445 = Compound Arithmetic op=OR(w711, w712, w762, w714) -> (w763:bool)
                  n446 = case shown="真" w763 {
                    frame False {
                    }
                    frame True {
                      n447 = local write "主界面选项"(enum32{"单选选项1", "单选选项2", "单选选项2 2", "单选选项2 3"}."单选选项1" ("主界面选项")) -> ()
                      n448 = local write "面板选择"(enum32{"读写参数", "版本读取", "其它诊断"}."读写参数" ("选项卡控件 2")) -> ()
                    }
                  }
                  n449 = property on="单选选项1" class="Bool (严格)"("Visible"=w763) -> ()  [unwired: 2 in, 2 out]
                }
                frame #2 {
                  n450 = control-ref of="单选选项2 2"() -> (w770:refnum<vi>)
                  n451 = control-ref of="单选选项2 3"() -> (w766:refnum<vi>)
                  n452 = control-ref of="单选选项2"() -> (w772:refnum<vi>)
                  n453 = control-ref of="单选选项1"() -> (w771:refnum<vi>)
                  n454 = local read "主界面选项"() -> (w775:enum32{"单选选项1", "单选选项2", "单选选项2 2", "单选选项2 3"})
                  n455 = Build Array(w771, w772, w770, w766) -> (w769:refnum<vi>[])
                  n456 = Delete From Array(array=w769, index=w775) -> (deleted portion=w773:refnum<vi>, array with subset deleted=w774:refnum<vi>[])  [unwired: 1 in]
                  n457 = property class="Bool (严格)"(reference=w773, "BoolText.TextColor"=u32 87470) -> ()  [unwired: 1 in, 2 out]
                  n458 = for {
                    tunnel: u32 16777215 -> [w777]
                    tunnel: w774 -> [w776] mode=indexing
                    n459 = property class="Bool (严格)"(reference=w776, "BoolText.TextColor"=w777) -> ()  [unwired: 1 in, 2 out]
                  }
                }
              }
            }
            frame #1 {
              # "项目信息"
              # "SOC"
              # "SOH"
              # "电池额定实际容量"
              # "车牌号"
              # "产品编号"
              # "电压个数"
              # "通道电压数"
              # "温度个数"
              # "电压起始值"
              # "温度起始值"
              # "配置文件版本"
              # "系统时钟"
              # "校正时钟"
              n460 = global read "功能码全局.vi" "主板项目信息5"() -> (w851:bool[])
              n461 = global read "功能码全局.vi" "主板项目信息6"() -> (w850:bool[])
              n462 = global read "功能码全局.vi" "主板项目信息7"() -> (w827:bool[])
              n463 = global read "功能码全局.vi" "主板项目信息4"() -> (w798:bool[])
              n464 = Index Array(array=w851) -> (element #1=w848:bool, element #2=w845:bool, element #3=w842:bool, element #4=w839:bool, element #5=w835:bool, element #6=w833:bool, element #7=w830:bool, element #8=w826:bool)  [unwired: 8 in]
              n465 = Index Array(array=w850) -> (element #1=w823:bool, element #2=w847:bool, element #3=w844:bool, element #4=w841:bool, element #5=w838:bool, element #6=w834:bool, element #7=w832:bool, element #8=w829:bool)  [unwired: 8 in]
              n466 = Index Array(array=w827) -> (element #1=w825:bool, element #2=w822:bool, element #3=w820:bool, element #4=w815:bool, element #5=w812:bool, element #6=w819:bool, element #7=w813:bool, element #8=w811:bool)  [unwired: 8 in]
              n467 = Index Array(array=w798) -> (element #6=w794:bool, element #7=w793:bool, element #8=w797:bool)  [unwired: 8 in, 5 out]
              n468 = Not(x=w797) -> (.not. x?=w796:bool)
              n469 = Not Or(1:w793, 2:w794) -> (0:w792:bool)
              n470 = Not Or(1:w847, 2:w848) -> (0:w810:bool)
              n471 = Not Or(1:w844, 2:w845) -> (0:w809:bool)
              n472 = Not Or(1:w841, 2:w842) -> (0:w808:bool)
              n473 = Not Or(1:w838, 2:w839) -> (0:w807:bool)
              n474 = Not Or(1:w834, 2:w835) -> (0:w806:bool)
              n475 = Not Or(1:w832, 2:w833) -> (0:w805:bool)
              n476 = Not Or(1:w829, 2:w830) -> (0:w804:bool)
              n477 = Not Or(1:w825, 2:w826) -> (0:w803:bool)
              n478 = Not Or(1:w819, 2:w820) -> (0:w801:bool)
              n479 = Not Or(1:w811, 2:w812) -> (0:w799:bool)
              n480 = Not Or(1:w813, 2:w815) -> (0:w800:bool)
              n481 = Not Or(1:w822, 2:w823) -> (0:w802:bool)
              n482 = Compound Arithmetic op=OR(w796, w810, w809, w808, w807, w806, w805, w804, w803, w802, w801, w800, w799) -> (w791:bool)
              "项目信息结果" <- w791
